vi "test Source Separated.vi"(8 "error in":errorcluster, 11 "TestCase in":refnum<class "Communication Bus Template Unit Tests.lvclass">) -> (0 "error out":errorcluster, 3 "TestCase out":refnum<class "Communication Bus Template Unit Tests.lvclass">)   [LabVIEW 2020, in "Communication Bus Template Unit Tests.lvclass"]
uses:
  Communication Bus Template Unit Tests.lvclass
  C:/Program Files (x86)/National Instruments/LabVIEW 2020/vi.lib/addons/_JKI Toolkits/VI Tester/TestCase.llb/TestCase.lvclass
  <vilib>/addons/_JKI Toolkits/VI Tester/TestCase.llb/TestCase.lvclass
  niveristand-custom-device-testing-tools/VeriStandTestUtilities/VeriStandTestUtilities.lvlib
  C:/Git/niveristand-ballard-arinc429-custom-device/Source/Custom Device/Tests/Unit/Communication Bus Template Unit Tests/Communication Bus Template Unit Tests.lvclass
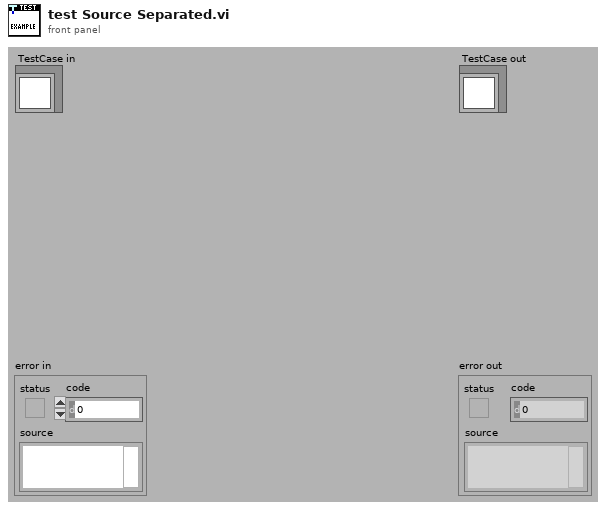
[diagram p1: front panel]
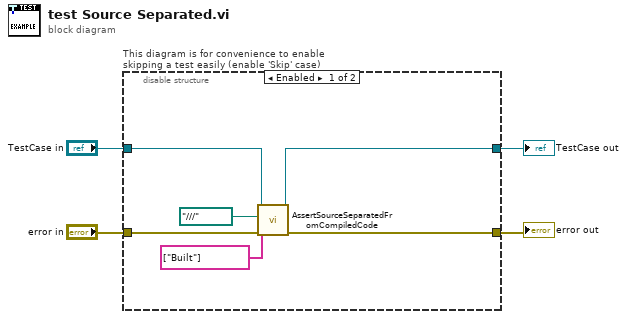
[diagram p0: block diagram]
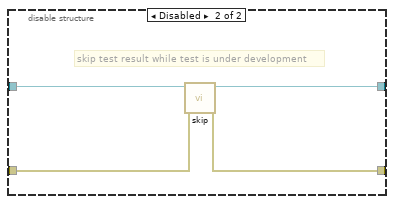
[diagram p2: hidden frame]
diagram:
  n1 = disable-structure "This diagram is for convenience to enable skipping a test easily (enable 'Skip' case)" shown="Enabled" {
    disable-tunnel: "TestCase in" -> [w8 w14]
    disable-tunnel: [w7 w12] -> w1
    disable-tunnel: [w9 w13] -> w3
    disable-tunnel: "error in" -> [w10 w11]
    frame Enabled {
      n2 = call "AssertSourceSeparatedFromCompiledCode.vi"("error in"=w10, "folders to exclude"=string[] ["Built"], "search path"=path "../../../..", "TestCase in"=w8) -> ("error out"=w9:errorcluster, "TestCase out"=w7:refnum<class "Communication Bus Template Unit Tests.lvclass">)  [unwired: 6 in]
    }
    frame Disabled {
      # "skip test result while test is under development"
      n3 = call <vilib>:"skip.vi"("error in (no error)"=w11, "TestCase in"=w14) -> ("error out"=w13:errorcluster, "TestCase out"=w12:refnum<class "Communication Bus Template Unit Tests.lvclass">)  [unwired: 8 in]
    }
  }
  "error out" <- w3
  "TestCase out" <- w1
